vi "CreateControl.vi"(0 "Owner":refnum<vi>, 1 "Type":T1, 2 "Array":bool, 3 "Label.Text":string, 4 "TypeDef":path, 5 "error in":errorcluster, 6 "AppRef":refnum<vi>, 7 "position/next to":cluster{"Horizontal":i16, "Vertical":i16}) -> (14 "reference out":refnum<vi>, 19 "error out":errorcluster)   [LabVIEW 2020, in "G#IDE.lvlib" / "ScriptingLib.lvlib"]
uses:
  ScriptingLib.lvlib
  DataTypes.ctl
  <vilib>/Utility/miscctls.llb/LVPointTypeDef.ctl
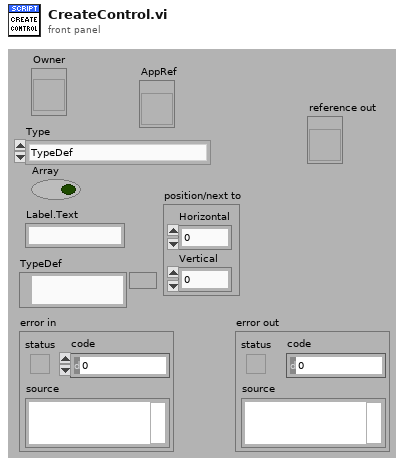
[diagram p1: front panel]
types:
  T1 = typedef "G#IDE.lvlib/ScriptingLib.lvlib/DataTypes.ctl" = enum16{"TypeDef", "I8", "I16", "I32", "I64", "U8", "U16", "U32", "U64", "SGL", "DBL", "EXT", "CSG", "CDB", "CXT", "ENUMU8", "ENUMU16", "ENUMU32", "BOOL", "STRING", "PATH", "PICT", "DAQ Channel Name", "CLUSTER", "VARIANT", "WAVEFORM", "DIGITAL WAVEFORM", "Automation REFNUM", "VI REFNUM", "LVCLASS", "CTL REFNUM", "TCP REFNUM", "OCC REFNUM", "QUEUE REFNUM", "DVR REFNUM", "Unknown", "Byte Stream File REFNUM", ".NET REFNUM", "Event Callback REFNUM", "Menu REFNUM", "App REFNUM", "UDP REFNUM", "IrDA REFNUM", "DataSocket REFNUM", "Bluetooth REFNUM", "Notifier REFNUM", "Semaphore REFNUM", "Rendevouz REFNUM", "VISA Resource", "IVI Logical Name"}
  T2 = typedef "LVPointTypeDef.ctl" = cluster{"Horizontal":i16, "Vertical":i16}
  T3 = enum32{"Extended Precision", "Double Precision", "Single Precision", "Long", "Word", "Byte", "Unsigned Long", "Unsigned Word", "Unsigned Byte", "Complex Extended", "Complex Double", "Complex Single", "Quad", "Unsigned Quad", "Fixed-Point"}
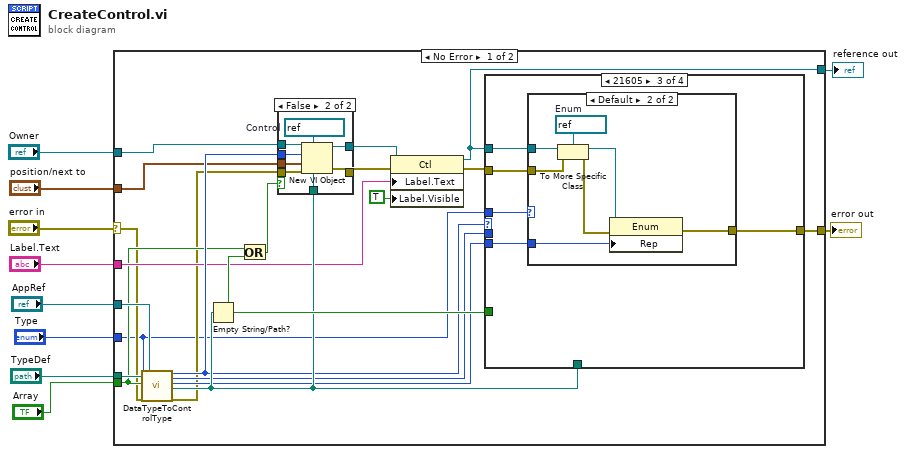
[diagram p0: block diagram]
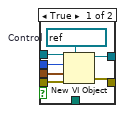
[diagram p2: hidden frame]
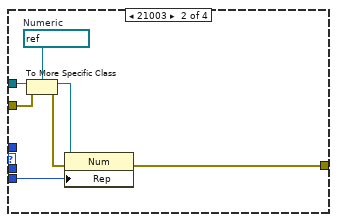
[diagram p4: hidden frame]
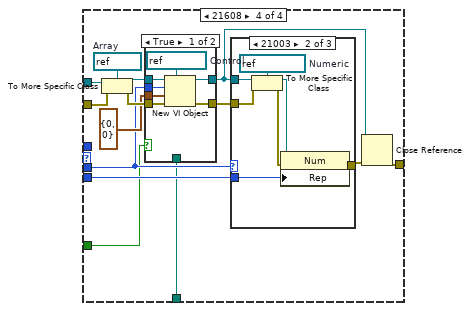
[diagram p6: hidden frame]
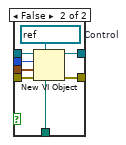
[diagram p7: hidden frame]
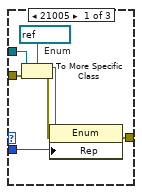
[diagram p8: hidden frame]
diagram:
  n1 = case shown="No Error" "error in" {
    selector: "error in" -> [w13 w112]
    tunnel: [w25 _] -> w10
    tunnel: "TypeDef" -> [w23 _]
    tunnel: "Type" -> [w11 _]
    tunnel: "AppRef" -> [w22 _]
    tunnel: "Owner" -> [w18 _]
    tunnel: "position/next to" -> [w17 _]
    tunnel: [w16 w112] -> w4
    tunnel: "Label.Text" -> [w15 _]
    tunnel: "Array" -> [w14 _]
    frame No Error {
      n2 = call "DataTypeToControlType.vi"("Type"=w11, "TypeDef"=w23, "Array"=w14, "error in"=w13, "AppRef"=w22) -> ("ControlStyle"=w21:u32, "InnerControlStyle"=w20:u32, "Representation"=w19:T3, "TypeDefOut"=w24:path, "error out"=w12:errorcluster)  [unwired: 9 in, 1 out]
      n3 = Empty String/Path?(string/path=w24) -> (empty?=w28:bool)
      n4 = Or(x=w14, y=w28) -> (x .or. y?=w29:bool)
      n5 = case shown="False" w29 {
        tunnel: w17 -> [w38 w46]
        tunnel: w18 -> [w37 w45]
        tunnel: w12 -> [w36 w44]
        tunnel: [w34 w42] -> w31
        tunnel: [w33 w41] -> w30
        tunnel: w21 -> [w32 w40]
        tunnel: w24 -> [_ w39]
        frame True {
          w35 = refnum<vi> refnum  # Control
          n6 = New VI Object(vi object class=w35, owner refnum=w37, style=w32, position/next to=w38, 8:w36) -> (object refnum=w33:refnum<vi>, 0:w34:errorcluster)  [unwired: 3 out]
        }
        frame False {
          w43 = refnum<vi> refnum  # Control
          n7 = New VI Object(vi object class=w43, owner refnum=w45, style=w40, position/next to=w46, 6:w39, 8:w44) -> (object refnum=w41:refnum<vi>, 0:w42:errorcluster)  [unwired: 2 out]
        }
      }
      n8 = property class="Ctl"(reference=w30, error in=w31, "Label.Text"=w15, "Label.Visible"=TRUE) -> (reference out=w25:refnum<vi>, error out=w26:errorcluster)
      n9 = case shown="21605" w21 {
        tunnel: w19 -> [_ w51 w59 w73]
        tunnel: w26 -> [w47 w50 w58 w80]
        tunnel: w25 -> [_ w49 w57 w79]
        tunnel: [w47 w48 w56 w72] -> w16
        tunnel: w20 -> [_ _ _ w75]
        tunnel: w28 -> [_ _ _ w69]
        tunnel: w24 -> [_ _ _ w68]
        tunnel: w11 -> [_ _ w55 _]
        frame Default {
        }
        frame 21003 {
          w54 = refnum<vi> refnum  # Numeric
          n10 = To More Specific Class(target class=w54, reference=w49, error in=w50) -> (specific class reference=w52:refnum<vi>, error out=w53:errorcluster)
          n11 = property class="Num"(reference=w52, error in=w53, "Rep"=w51) -> (error out=w48:errorcluster)  [unwired: 1 out]
        }
        frame 21605 {
          n12 = case shown="Default" w55 {
            tunnel: w59 -> [_ w64]
            tunnel: w58 -> [w60 w63]
            tunnel: w57 -> [_ w62]
            tunnel: [w60 w61] -> w56
            frame "TypeDef" {
            }
            frame Default {
              w67 = refnum<vi> refnum  # Enum
              n13 = To More Specific Class(target class=w67, reference=w62, error in=w63) -> (specific class reference=w65:refnum<vi>, error out=w66:errorcluster)
              n14 = property class="Enum"(reference=w65, error in=w66, "Rep"=w64) -> (error out=w61:errorcluster)  [unwired: 1 out]
            }
          }
        }
        frame 21608 {
          w81 = refnum<vi> refnum  # Array
          n15 = To More Specific Class(target class=w81, reference=w79, error in=w80) -> (specific class reference=w77:refnum<vi>, error out=w78:errorcluster)
          n16 = case shown="True" w69 {
            tunnel: w78 -> [w88 w96]
            tunnel: w77 -> [w87 w95]
            tunnel: T2 {"Horizontal"=0, "Vertical"=0} ("relative position/next to refnum") -> [w85 w93]
            tunnel: w75 -> [w84 w92]
            tunnel: [w83 w91] -> w74
            tunnel: [w82 w90] -> w70
            tunnel: w68 -> [_ w89]
            frame True {
              w86 = refnum<vi> refnum  # Control
              n17 = New VI Object(vi object class=w86, owner refnum=w87, style=w84, position/next to=w85, 8:w88) -> (object refnum=w82:refnum<vi>, 0:w83:errorcluster)  [unwired: 3 out]
            }
            frame False {
              w94 = refnum<vi> refnum  # Control
              n18 = New VI Object(vi object class=w94, owner refnum=w95, style=w92, position/next to=w93, 6:w89, 8:w96) -> (object refnum=w90:refnum<vi>, 0:w91:errorcluster)  [unwired: 2 out]
            }
          }
          n19 = case shown="21003" w75 {
            tunnel: w74 -> [w100 w107 w111]
            tunnel: w70 -> [w99 w106 _]
            tunnel: [w97 w105 w111] -> w71
            tunnel: w73 -> [w98 w104 _]
            frame 21005 {
              w103 = refnum<vi> refnum  # Enum
              n20 = To More Specific Class(target class=w103, reference=w99, error in=w100) -> (specific class reference=w101:refnum<vi>, error out=w102:errorcluster)
              n21 = property class="Enum"(reference=w101, error in=w102, "Rep"=w98) -> (error out=w97:errorcluster)  [unwired: 1 out]
            }
            frame 21003 {
              w110 = refnum<vi> refnum  # Numeric
              n22 = To More Specific Class(target class=w110, reference=w106, error in=w107) -> (specific class reference=w108:refnum<vi>, error out=w109:errorcluster)
              n23 = property class="Num"(reference=w108, error in=w109, "Rep"=w104) -> (error out=w105:errorcluster)  [unwired: 1 out]
            }
            frame Default {
            }
          }
          n24 = Close Reference(reference=w70, error in (no error)=w71) -> (error out=w72:errorcluster)
        }
      }
    }
    frame Error {
    }
  }
  "error out" <- w4
  "reference out" <- w10
